vi "ReadFromTXT.vi"   [LabVIEW 2019]
uses:
  DashboardGlobals.vi
  <vilib>/Utility/file.llb/Read Delimited Spreadsheet (string).vi
  <vilib>/Rock Robotics/Network Tables/NT Write Numeric Array.vi
  <vilib>/Rock Robotics/Network Tables/NT Write String Array.vi
  <vilib>/Rock Robotics/Network Tables/NT Write Boolean Array.vi
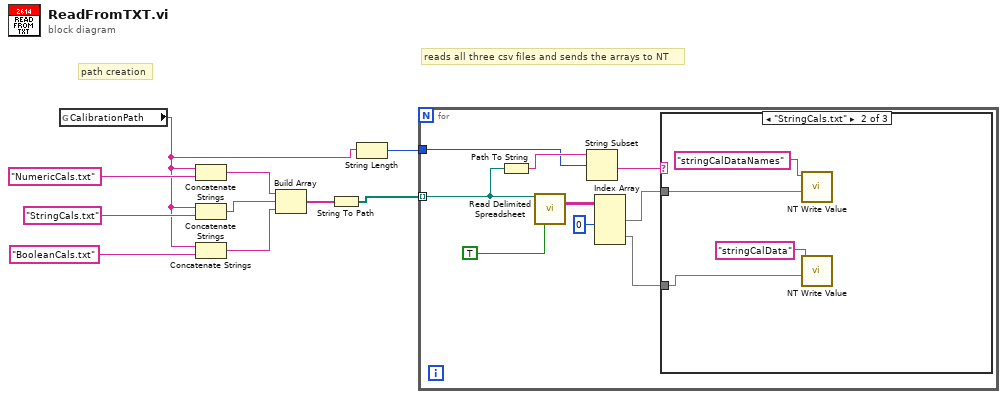
[diagram p0: block diagram]
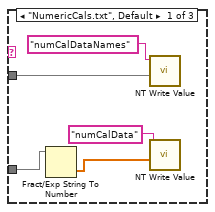
[diagram p2: hidden frame]
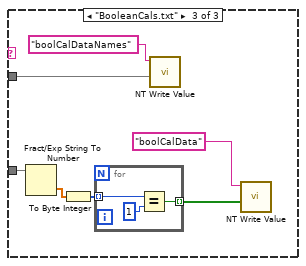
[diagram p3: hidden frame]
diagram:
  # "reads all three csv files and sends the arrays to NT"
  # "path creation"
  n1 = global read "DashboardGlobals.vi" "CalibrationPath"() -> (w1:string)
  n2 = Concatenate Strings(w1, "NumericCals.txt" ("string")) -> (w3:string)
  n3 = Concatenate Strings(w1, "StringCals.txt" ("string")) -> (w7:string)
  n4 = Concatenate Strings(w1, "BooleanCals.txt" ("string")) -> (w6:string)
  n5 = Build Array(w3, w7, w6) -> (w5:string[])
  n6 = String To Path(string=w5) -> (path=w4:path[])
  n7 = String Length(string=w1) -> (length=w2:i32)
  n8 = for {
    tunnel: w4 -> [w16] mode=indexing
    tunnel: w2 -> [w11]
    n9 = Path To String(path=w16) -> (string=w15:string)
    n10 = call-poly <vilib>:"Read Delimited Spreadsheet.vi"("file path (dialog if empty)"=w16, "transpose? (F)"=TRUE) -> ("all rows"=w19:string[][])  [unwired: 8 in, 5 out]
    n11 = String Subset(string=w15, offset (0)=w11) -> (substring=w14:string)  [unwired: 1 in]
    n12 = Index Array(array=w19, index (col) #1=0 ("disabled index (col)")) -> (element #1=w13:string[], element #2=w12:string[])  [unwired: 3 in]
    n13 = case shown="\"StringCals.txt\"" w14 {
      tunnel: w13 -> [w24 w28 w35]
      tunnel: w12 -> [w22 w25 w32]
      frame "NumericCals.txt", Default {
        n14 = Fract/Exp String To Number(string=w22) -> (number=w21:dbl[])  [unwired: 3 in, 1 out]
        n15 = call-poly <vilib>:"NT Write Value.vi"("String Array"=w24, "Name"="numCalDataNames") -> ()  [unwired: 9 in, 1 out]
        n16 = call-poly <vilib>:"NT Write Value.vi"("Numeric Array"=w21, "Name"="numCalData") -> ()  [unwired: 9 in, 1 out]
      }
      frame "StringCals.txt" {
        n17 = call-poly <vilib>:"NT Write Value.vi"("String Array"=w28, "Name"="stringCalDataNames") -> ()  [unwired: 9 in, 1 out]
        n18 = call-poly <vilib>:"NT Write Value.vi"("String Array"=w25, "Name"="stringCalData") -> ()  [unwired: 9 in, 1 out]
      }
      frame "BooleanCals.txt" {
        n19 = Fract/Exp String To Number(string=w32) -> (number=w31:dbl[])  [unwired: 3 in, 1 out]
        n20 = To Byte Integer(number=w31) -> (8bit integer=w30:i8[])
        n21 = for {
          tunnel: w30 -> [w38] mode=indexing
          tunnel: [w37] -> w29 mode=indexing
          n22 = Equal?(x=w38, y=i8 1) -> (x = y?=w37:bool)
        }
        n23 = call-poly <vilib>:"NT Write Value.vi"("String Array"=w35, "Name"="boolCalDataNames") -> ()  [unwired: 9 in, 1 out]
        n24 = call-poly <vilib>:"NT Write Value.vi"("Boolean Array"=w29, "Name"="boolCalData") -> ()  [unwired: 9 in, 1 out]
      }
    }
  }
